vi "emi_Defer Panel Updates ON(w.cursor).vi"(5 "VI Refnum(This VI)":refnum<vi>, 9 "error in (no error)":errorcluster) -> (6 "VI Refnum Out":refnum<vi>, 10 "error out":errorcluster)   [LabVIEW 2011]
doc: "Gets a vi panel refrence, sets defere panel update to true, close panel refrence.\n\nIf not VI Refnum in, the refrence of the vi where this funciton is used is employed, and subsequently closed. (If refrence not explisitly vired, it does not need to be closed)\n\nIf error: No action."
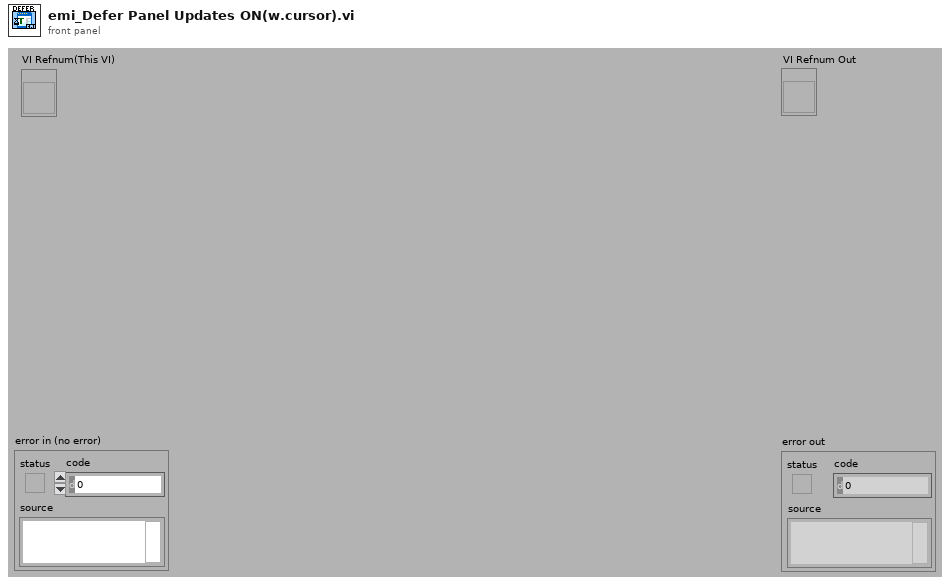
[diagram p1: front panel]
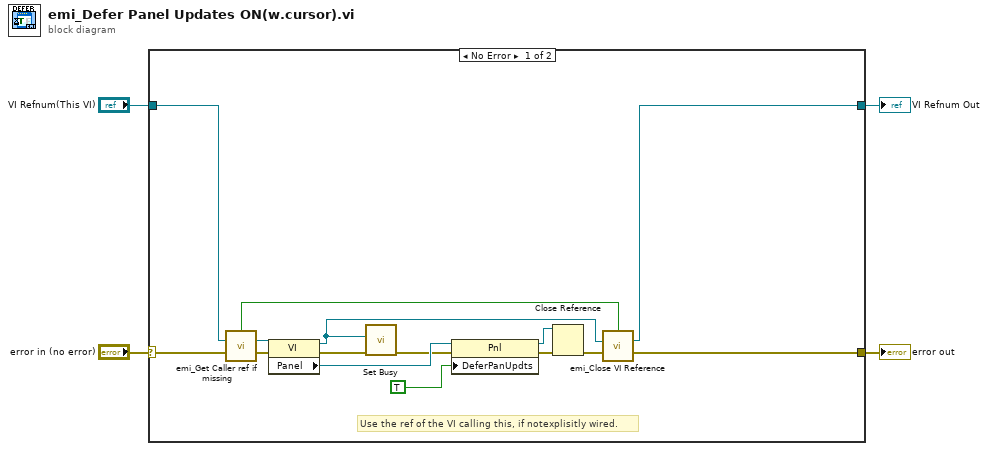
[diagram p0: block diagram]
diagram:
  n1 = case shown="No Error" "error in (no error)" {
    selector: "error in (no error)" -> [w14 w21]
    tunnel: [w12 w21] -> w3
    tunnel: "VI Refnum(This VI)" -> [w10 w20]
    tunnel: [w8 w20] -> w1
    frame No Error {
      # "Use the ref of the VI calling this, if notexplisitly wired."
      n2 = call "emi_Get Caller ref if missing.vi"("VI Refnum(Calling VI)"=w10, "error in (no error)"=w14) -> ("Ref Generated"=w15:bool, "VI Refnum Out"=w9:refnum<vi>, "error out"=w13:errorcluster)  [unwired: 11 in]
      n3 = property class="VI"(reference=w9, error in=w13) -> (reference out=w5:refnum<vi>, error out=w7:errorcluster, "Panel"=w18:refnum<vi>)
      n4 = call <vilib>:"Set Busy.vi"("error in (no error)"=w7, "VI reference (current VI)"=w5) -> ("error out"=w6:errorcluster)  [unwired: 8 in, 1 out]
      n5 = property class="Pnl"(reference=w18, error in=w6, "DeferPanUpdts"=TRUE ("Defer Panel Updates")) -> (reference out=w17:refnum<vi>, error out=w16:errorcluster)
      n6 = Close Reference(reference=w17, error in (no error)=w16) -> (error out=w11:errorcluster)
      n7 = call "emi_Close VI Reference.vi"("Close ref?(T)"=w15, "VI Refnum"=w5, "error in (no error)"=w11) -> ("VI Refnum Out"=w8:refnum<vi>, "error out"=w12:errorcluster)  [unwired: 11 in]
    }
    frame Error {
    }
  }
  "error out" <- w3
  "VI Refnum Out" <- w1
